vi "Auswerten.vi"(8 "LIN Ausgabetabelle":refnum<vi>, 9 "Komponente:":refnum<vi>, 10 "max. Flow Weighted Mean:":refnum<vi>) -> (0 "Konzentration Komponente":dbl, 1 "Komponente:":T1, 2 "max. Flow Weighted Mean:":T1, 3 "Konzentration FlowWeightedMean":dbl, 4 "Limit in ppm":dbl, 5 "[%]":dbl)   [LabVIEW 2020, in "EPA 1065.lvlib" / "HovaCAL Interference verificaton.lvlib"]
uses:
  HovaCAL Interference verificaton.lvlib
  <vilib>/Utility/miscctls.llb/LVRowAndColumnTypeDef.ctl
  Sprachverwaltung/Sprachverwaltung.lvlib
  Sprachverwaltung/FGV Aktion Tabelle zerlegen.ctl
  Aktion FGV Interference.ctl
  Visualisierungs Elemente/String - Ausgabefeld.ctl
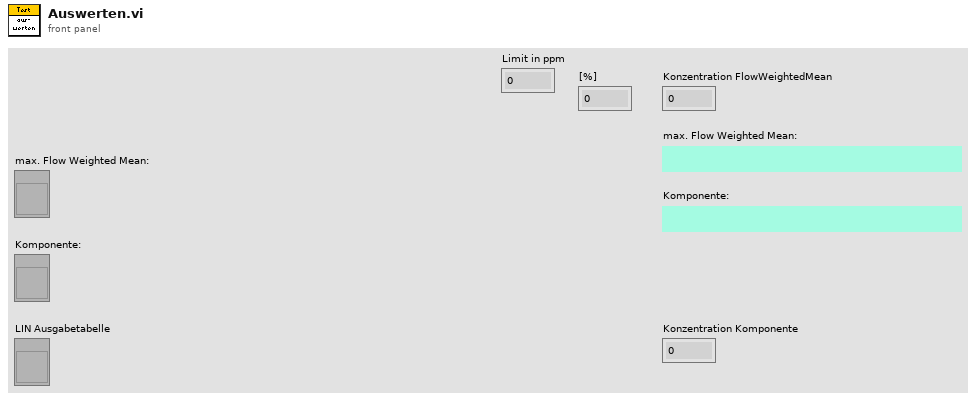
[diagram p1: front panel]
types:
  T1 = typedef "String - Ausgabefeld.ctl" = string
  T2 = typedef "EPA 1065.lvlib/HovaCAL Interference verificaton.lvlib/Aktion FGV Interference.ctl" = enum16{"Lesen", "TestKonfig", "TestSetting", "Einheiten", "Ergebnis", "Laden", "Tabelle", "Speichern", "löschen"}
  T3 = typedef "Sprachverwaltung.lvlib/FGV Aktion Tabelle zerlegen.ctl" = enum16{"laden", "vereinzeln", "speichern"}
  T4 = typedef "LVRowAndColumnTypeDef.ctl" = cluster{"Row":i32, "Column":i32}
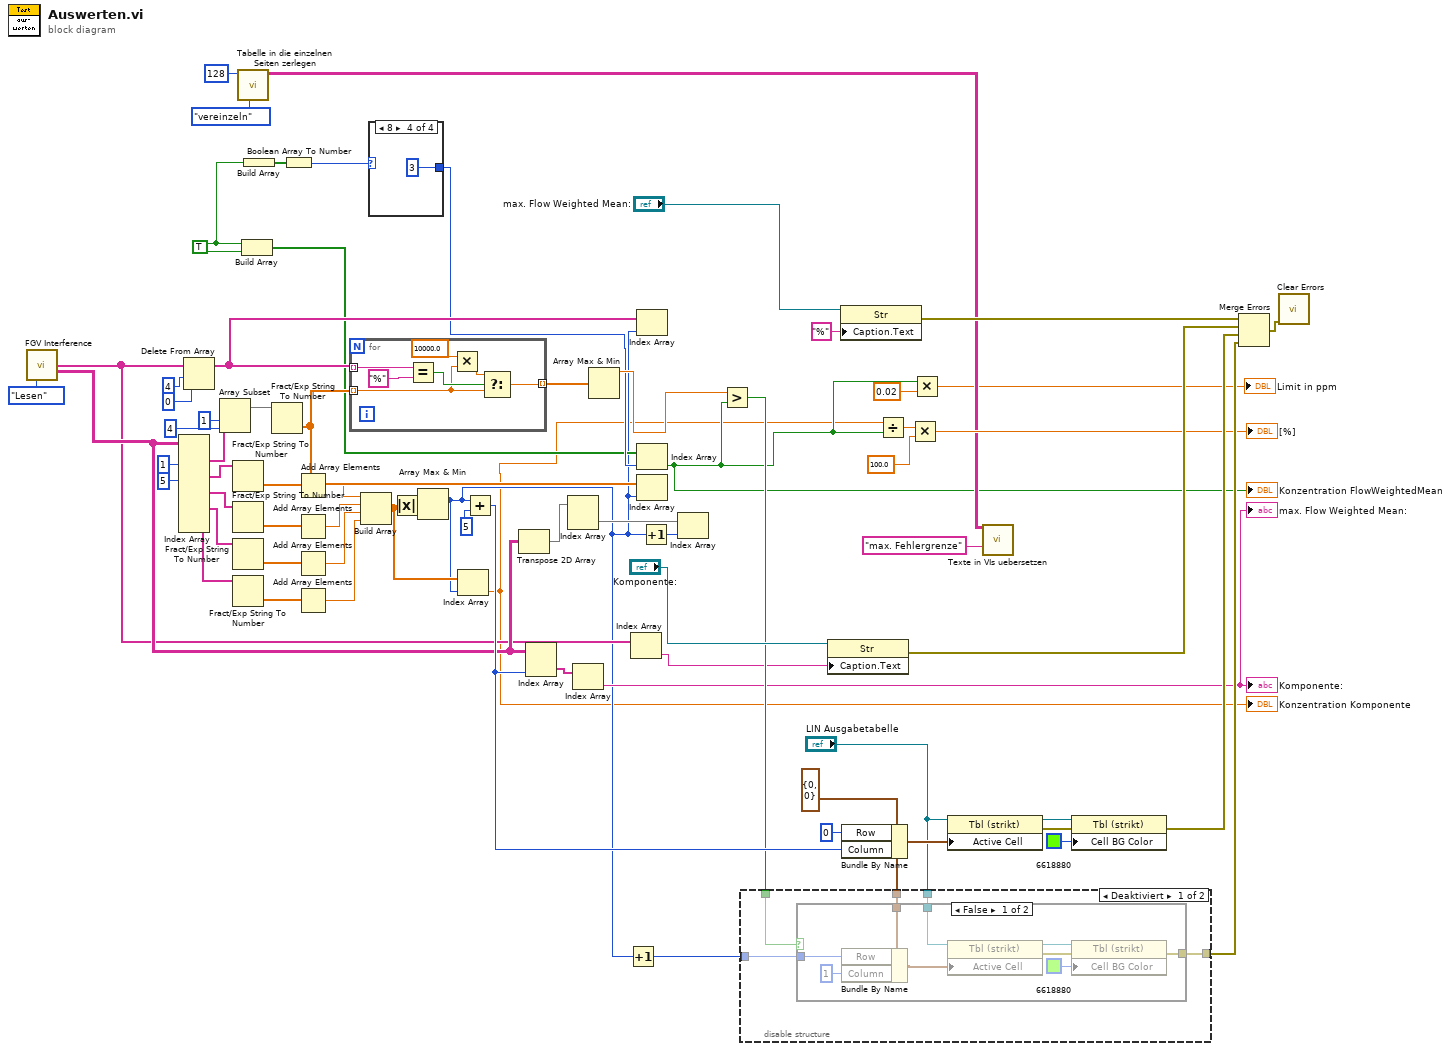
[diagram p0: block diagram]
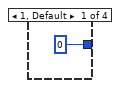
[diagram p2: hidden frame]
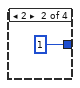
[diagram p3: hidden frame]
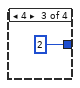
[diagram p4: hidden frame]
diagram:
  w1 = TRUE
  w65 = T4 {"Row"=0, "Column"=0} ("Aktive Zelle:Aktive Zelle")
  n1 = call "FGV Interference.vi"("Aktion FGV Interference"=Aktion_FGV_Interference."Lesen") -> ("Einheiten"=w13:string[], "Tabelle"=w21:T1[][])  [unwired: 9 in, 4 out]
  n2 = Index Array(array=w21, index (col) #1=1 ("Deaktivierter Index (Spalte)"), index (col) #2=5 ("Index (Spalte)")) -> (element #1=w42:T1[], element #2=w43:T1[], element #3=w44:T1[], element #4=w45:T1[], element #5=w7:T1[])  [unwired: 8 in]
  n3 = Delete From Array(array=w13, length=4 ("Länge"), index=0 ("Index")) -> (array with subset deleted=w46:string[])  [unwired: 1 out]
  n4 = Array Subset(array=w42, index=1 ("Index"), length=4 ("Länge")) -> (w38:T1[])
  n5 = Fract/Exp String To Number(string=w43) -> (number=w11:dbl[])  [unwired: 3 in, 1 out]
  n6 = Fract/Exp String To Number(string=w44) -> (number=w10:dbl[])  [unwired: 3 in, 1 out]
  n7 = Fract/Exp String To Number(string=w45) -> (number=w9:dbl[])  [unwired: 3 in, 1 out]
  n8 = Fract/Exp String To Number(string=w7) -> (number=w8:dbl[])  [unwired: 3 in, 1 out]
  n9 = call "Tabelle in die einzelnen Seiten zerlegen.vi"("Aktion"=FGV_Aktion_Tabelle_zerlegen."vereinzeln", "Index (Seite)"=128) -> ("Sprachliste"=w29:string[][])  [unwired: 7 in, 2 out]
  n10 = Build Array(w1, w1) -> (w17:bool[])
  n11 = Build Array(w1) -> (w20:bool[])
  n12 = Fract/Exp String To Number(string=w38) -> (number=w51:dbl[])  [unwired: 3 in, 1 out]
  n13 = Boolean Array To Number(Boolean array=w20) -> (number=w19:u32)
  n14 = Add Array Elements(numeric array=w11) -> (sum=w47:dbl)
  n15 = Add Array Elements(numeric array=w10) -> (sum=w48:dbl)
  n16 = Add Array Elements(numeric array=w9) -> (sum=w49:dbl)
  n17 = Add Array Elements(numeric array=w8) -> (sum=w6:dbl)
  n18 = for {
    tunnel: w46 -> [w74] mode=indexing
    tunnel: w51 -> [w73] mode=indexing
    tunnel: [w72] -> w12 mode=indexing
    n19 = Equal?(x=w74, y="%") -> (x = y?=w77:bool)
    n20 = Multiply(x=10000.0, y=w73) -> (x*y=w76:dbl)
    n21 = Select(t=w76, s=w77, f=w73) -> (s? t:f=w72:dbl)
  }
  n22 = Build Array(w47, w48, w49, w6) -> (w5:dbl[])
  n23 = case shown="8" w19 {
    tunnel: [0 1 2 3] -> w18
    frame 1, Default {
    }
    frame 2 {
    }
    frame 4 {
    }
    frame 8 {
    }
  }
  n24 = Absolute Value(x=w5) -> (abs(x)=w4:dbl[])
  n25 = Array Max & Min(array=w4) -> (max index (indices)=w3:i32)  [unwired: 3 out]
  n26 = Index Array(array=w5, index=w3) -> (element=w2:dbl)
  "Konzentration Komponente" <- w2
  n27 = Add(x=w3, y=5) -> (x+y=w63:i32)
  n28 = Transpose 2D Array(2D array=w21) -> (transposed array=w39:T1[][])
  n29 = Index Array(array=w21, index (col)=w63) -> (element=w50:T1[])  [unwired: 1 in]
  n30 = Index Array(array=w39) -> (element=w52:T1[])  [unwired: 2 in]
  n31 = Index Array(array=w50) -> (element=→"max. Flow Weighted Mean:" →"Komponente:":T1)  [unwired: 1 in]
  n32 = Array Max & Min(array=w12) -> (max value=w33:dbl)  [unwired: 3 out]
  n33 = Increment(x=w3) -> (x+1=w35:i32)
  n34 = Index Array(array=w13) -> (element=w28:string)  [unwired: 1 in]
  n35 = Index Array(array=w46, index=w3) -> ()  [unwired: 1 out]
  n36 = Index Array(array=w17, index=w18) -> (element=w16:bool)
  "Konzentration FlowWeightedMean" <- w16
  n37 = Index Array(array=w51, index=w3) -> ()  [unwired: 1 out]
  n38 = Increment(x=w3) -> (x+1=w34:i32)
  n39 = Index Array(array=w52, index=w34) -> ()  [unwired: 1 out]
  n40 = Greater?(x=w33, y=w16) -> (0:w32:bool)
  n41 = disable-structure shown="Deaktiviert" {
    disable-tunnel: [w87 _] -> w70
    disable-tunnel: w65 -> [w86 _]
    disable-tunnel: "LIN Ausgabetabelle" -> [w85 _]
    disable-tunnel: w35 -> [w84 _]
    disable-tunnel: w32 -> [w83 _]
    frame Disabled {
      n42 = case shown="False" w83 {
        tunnel: [w96 _] -> w87
        tunnel: w86 -> [w93 _]
        tunnel: w85 -> [w91 _]
        tunnel: w84 -> [w88 _]
        frame False {
          n43 = Bundle By Name(cluster=w93, "Row"=w88, "Column"=1) -> (w92:T4)
          n44 = property on="Eigenschaftsknoten" class="Tbl (strikt)"(reference=w91, "Active Cell"=w92) -> (reference out=w95:refnum<vi>, error out=w90:errorcluster)  [unwired: 1 in]
          n45 = property on="Eigenschaftsknoten" class="Tbl (strikt)"(reference=w95, error in=w90, "Cell BG Color"=u32 6618880) -> (error out=w96:errorcluster)  [unwired: 1 out]
        }
        frame True {
        }
      }
    }
    frame Enabled {
    }
  }
  n46 = property on="Eigenschaftsknoten" class="Str"(reference="Komponente:", "Caption.Text"=w28) -> (error out=w68:errorcluster)  [unwired: 1 in, 1 out]
  n47 = property on="Eigenschaftsknoten" class="Str"(reference="max. Flow Weighted Mean:", "Caption.Text"="%" ("Untertitel.Text")) -> (error out=w67:errorcluster)  [unwired: 1 in, 1 out]
  n48 = Bundle By Name(cluster=w65, "Row"=0, "Column"=w63) -> (w71:T4)
  n49 = Divide(x=w2, y=w16) -> (x/y=w26:dbl)
  n50 = Multiply(x=w26, y=100.0) -> (x*y=→"[%]":dbl)
  n51 = Multiply(x=w16, y=0.02) -> (x*y=→"Limit in ppm":dbl)
  n52 = property on="Eigenschaftsknoten" class="Tbl (strikt)"(reference="LIN Ausgabetabelle", "Active Cell"=w71) -> (reference out=w60:refnum<vi>, error out=w59:errorcluster)  [unwired: 1 in]
  n53 = call "Texte in VIs uebersetzen.vi"("Sprachliste"=w29, "String zum Übersetzen"="max. Fehlergrenze" ("String - Ausgabefeld")) -> ()  [unwired: 9 in, 5 out]
  n54 = property on="Eigenschaftsknoten" class="Tbl (strikt)"(reference=w60, error in=w59, "Cell BG Color"=u32 6618880) -> (error out=w69:errorcluster)  [unwired: 1 out]
  n55 = Merge Errors(w67, w68, w69, w70) -> (w66:errorcluster)
  n56 = call <vilib>:"Clear Errors.vi"("error in (no error)"=w66) -> ()  [unwired: 5 in, 2 out]
